vi "Interpolation_3Wheel.vi"(8 "error in (no error)":errorcluster, 10 "Cluster":cluster{"UD(mm)":dbl, "Vcmd":dbl}, 11 "KNR in":T2) -> (0 "error out":errorcluster, 2 "output cluster":T1, 3 "KNR out":T2)   [LabVIEW 2013]
uses:
  <userlib>/KNR OS 3.0 LabVIEW Toolkit/Type Definition/KNR3 Reference.ctl
  <userlib>/_FPGA Interface Advanced Tools/FPGA Interface Base/FPGA Interface Base.lvclass
  <userlib>/KNR OS 3.0 LabVIEW Toolkit/Type Definition/Resource.ctl
  Global.vi
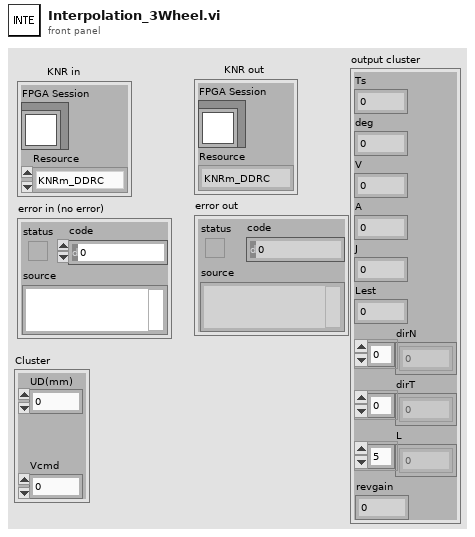
[diagram p1: front panel]
types:
  T1 = cluster{"Ts":dbl, "deg":dbl, "V":dbl, "A":dbl, "J":dbl, "Lest":dbl, "dirN":i32[], "dirT":dbl[], "L":dbl[], "revgain":dbl}
  T2 = typedef "KNR3 Reference.ctl" = cluster{"FPGA Session":refnum<class "FPGA Interface Base.lvclass">, "Resource":T3}
  T3 = typedef "Resource.ctl" = enum16{"KNRm_DDRC", "KNRm_DDDD", "KNRm_DDDR", "KNRm_DDDC", "KNR"}
  T4 = typedef "DC Motor Port.ctl" = u16
  T5 = cluster{"MM2DEG":dbl, "PLS2DEG":dbl, "Ts":dbl, "Tcnt":i32, "fs":i32, "Vmax":dbl, "Jmax":dbl, "N_Delay":i32, "C_port":T4, "KNRPLS":dbl}
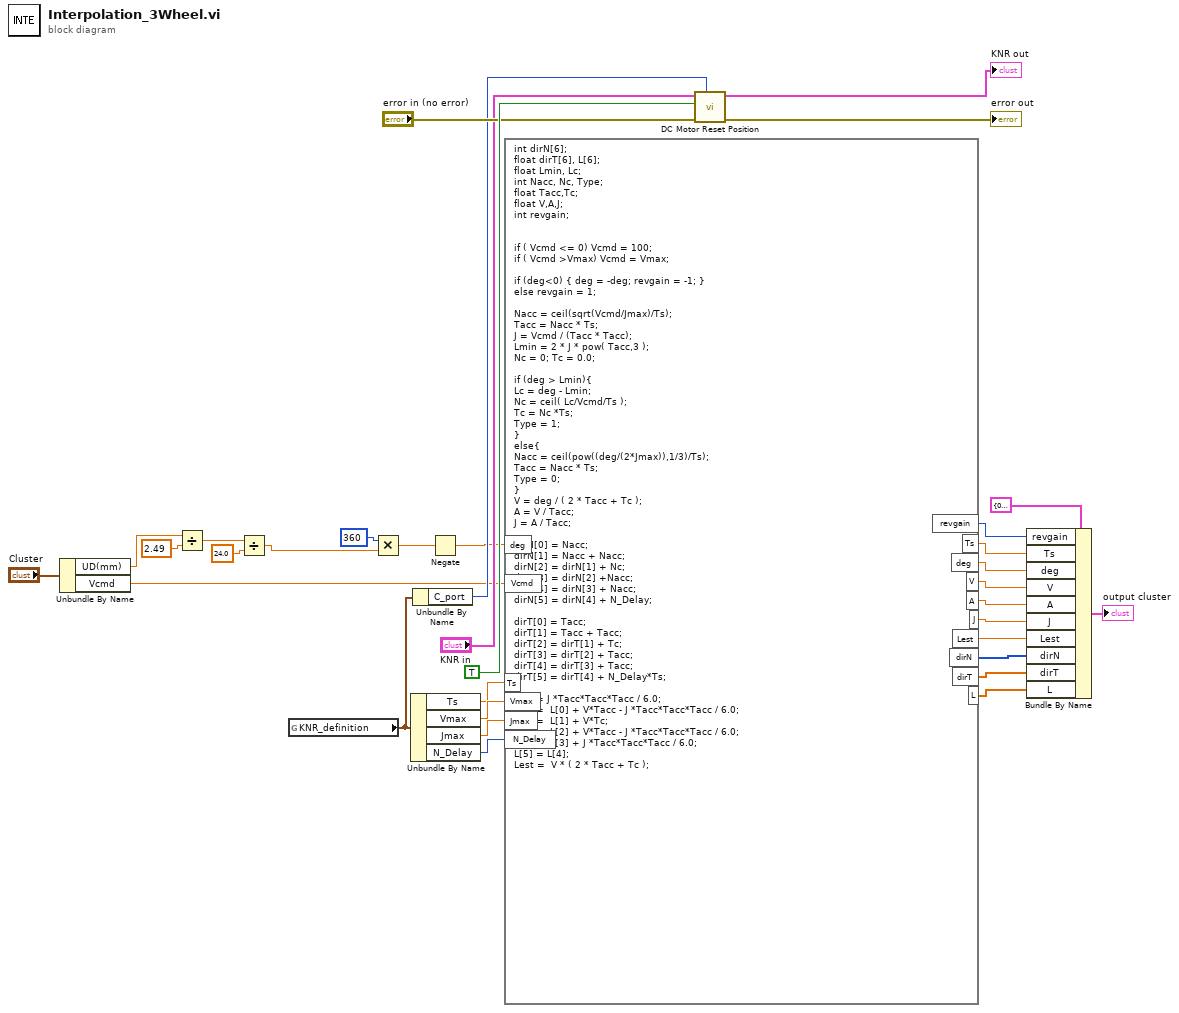
[diagram p0: block diagram]
diagram:
  n1 = Unbundle By Name("Cluster") -> ("UD(mm)"=w6:dbl, "Vcmd"=w14:dbl)
  n2 = Divide(x=w6, y=2.49) -> (x/y=w5:dbl)
  n3 = Divide(x=w5, y=24.0) -> (x/y=w1:dbl)
  n4 = global read "Global.vi" "KNR_definition"() -> (w29:T5)
  n5 = Multiply(x=360, y=w1) -> (x*y=w3:dbl)
  n6 = Unbundle By Name(w29) -> ("Ts"=w26:dbl, "Vmax"=w28:dbl, "Jmax"=w27:dbl, "N_Delay"=w25:i32)
  n7 = Unbundle By Name(w29) -> ("C_port"=w30:T4)
  n8 = Negate(x=w3) -> (-x=w2:dbl)
  n9 = formula code="int dirN[6];\nfloat dirT[6], L[6];\nfloat Lmin, Lc;\nint Nacc, Nc, Type;\nfloat Tacc,Tc;\nfloat V,A,J;\nint revgain;\n\n\nif ( Vcmd <= 0) Vcmd = 100;\nif ( Vcmd >Vmax) Vcmd = Vmax;\n\nif (deg<0) { deg = -deg; revgain = -1; }\nelse revgain = 1;\n\nNacc = ceil(sqrt(Vcmd/Jmax)/Ts);\nTacc = Nacc * Ts;\nJ = Vcmd / (Tacc * Tacc);\nLmin = 2 * J * pow( Tacc,3 ); \nNc = 0; Tc = 0.0;\n\nif (deg > Lmin){\nLc = deg - Lmin;\nNc = ceil( Lc/Vcmd/Ts );\nTc = Nc *Ts;\nType = 1;\n}\nelse{\nNacc = ceil(pow((deg/(2*Jmax)),1/3)/Ts);\nTacc = Nacc * Ts;\nType = 0;\n}\nV = deg / ( 2 * Tacc + Tc );\nA = V / Tacc;\nJ = A / Tacc;\n\ndirN[0] = Nacc;\ndirN[1] = Nacc + Nacc;\ndirN[2] = dirN[1] + Nc;\ndirN[3] = dirN[2] +Nacc;\ndirN[4] = dirN[3] + Nacc;\ndirN[5] = dirN[4] + N_Delay;\n\ndirT[0] = Tacc;\ndirT[1] = Tacc + Tacc;\ndirT[2] = dirT[1] + Tc;\ndirT[3] = dirT[2] + Tacc;\ndirT[4] = dirT[3] + Tacc;\ndirT[5] = dirT[4] + N_Delay*Ts;\n\nL[0] = J *Tacc*Tacc*Tacc / 6.0;\nL[1] =  L[0] + V*Tacc - J *Tacc*Tacc*Tacc / 6.0;\nL[2] =  L[1] + V*Tc;\nL[3] =  L[2] + V*Tacc - J *Tacc*Tacc*Tacc / 6.0;\nL[4] =  L[3] + J *Tacc*Tacc*Tacc / 6.0;\nL[5] = L[4];\nLest =  V * ( 2 * Tacc + Tc );"("Vcmd"=w14, "Vmax"=w28, "Jmax"=w27, "Ts"=w26, "N_Delay"=w25, "deg"=w2) -> ("deg"=w23:dbl, "Lest"=w19:dbl, "dirN"=w18:i32[], "V"=w22:dbl, "A"=w21:dbl, "J"=w20:dbl, "Ts"=w17:dbl, "dirT"=w16:dbl[], "L"=w15:dbl[], "revgain"=w8:i32)
  n10 = call <userlib>:"DC Motor Reset Position.vi"("Port (DS1)"=w30, "error in (no error)"="error in (no error)", "Reset(F)"=TRUE, "KNR in"="KNR in") -> ("error out"=→"error out":errorcluster, "KNR out"=→"KNR out":T2)  [unwired: 6 in]
  n11 = Bundle By Name(cluster=T1 {"Ts"=0.0, "deg"=0.0, "V"=0.0, "A"=0.0, "J"=0.0, "Lest"=0.0, "dirN"=[], "dirT"=[], "L"=[], "revgain"=0.0} ("Cluster 2"), "revgain"=w8, "Ts"=w17, "deg"=w23, "V"=w22, "A"=w21, "J"=w20, "Lest"=w19, "dirN"=w18, "dirT"=w16, "L"=w15) -> (→"output cluster":T1)
